vi "PID.vi"(6 "reinitialize? (F)":bool, 8 "dt (s)":dbl=-1.0 format="%#_13g", 11 "control":T2) -> (2 "output":dbl format="%.2f")   [LabVIEW 2019, in "my FPGA lib.lvlib" / "motor.lvclass"]
uses:
  motor.lvclass
  control/PID control.ctl
  <vilib>/addons/control/pid/pid.llb/PID (DBL).vi
  <vilib>/addons/control/pid/NI_PID_pid.lvlib
panel:
  in  "PID gains":T1={"proportional gain (Kc)"=1.0, "integral time (Ti, min)"=0.01, "derivative time (Td, min)"=0.0} {"derivative time (Td, min)" format="%.3f"; "integral time (Ti, min)" format="%.3f"; "proportional gain (Kc)" format="%.3f"}
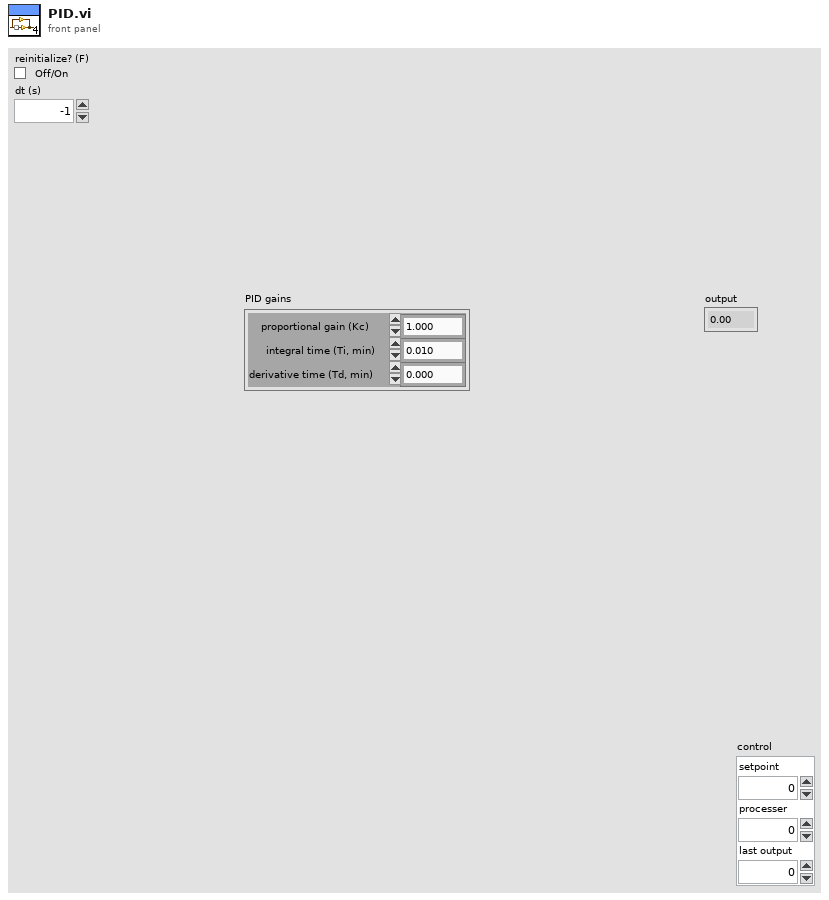
[diagram p1: front panel]
types:
  T1 = cluster{"proportional gain (Kc)":dbl, "integral time (Ti, min)":dbl, "derivative time (Td, min)":dbl}
  T2 = typedef "my FPGA lib.lvlib/motor.lvclass/PID control.ctl" = cluster{"setpoint":dbl, "processer":dbl, "last output":dbl}
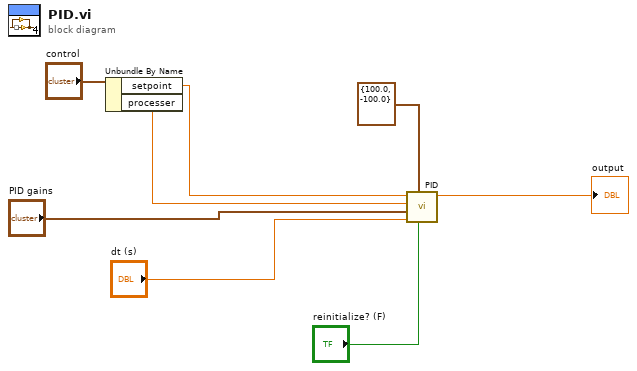
[diagram p0: block diagram]
diagram:
  n1 = Unbundle By Name("control") -> ("setpoint"=w6:dbl, "processer"=w5:dbl)
  n2 = call-poly <vilib>:"PID.vi"("reinitialize? (F)"="reinitialize? (F)", "output range"=cluster{"output high":dbl, "output low":dbl} {"output high"=100.0, "output low"=-100.0}, "dt (s)"="dt (s)", "PID gains"="PID gains", "process variable"=w5, "setpoint"=w6) -> ("output"=→"output":dbl)  [unwired: 4 in, 1 out]
